vi "Get(X,Y)2.vi"(2 "[IN] index of (X,Y)":i32, 3 "[IN] Array coordi\nnates (X,Y) in Frame":dbl[](array[numeric])) -> (0 "[OUT] Y":dbl, 1 "[OUT] X":dbl)   [LabVIEW 2013]
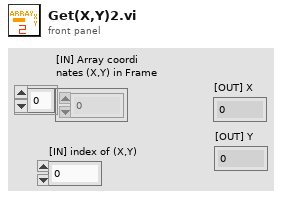
[diagram p1: front panel]
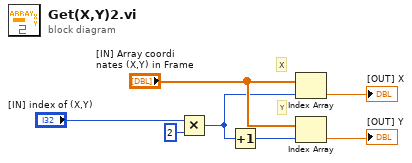
[diagram p0: block diagram]
diagram:
  # "Y"
  # "X"
  n1 = Multiply(x="[IN] index of (X,Y)", y=2) -> (x*y=w1:i32)
  n2 = Increment(x=w1) -> (x+1=w4:i32)
  n3 = Index Array(array="[IN] Array coordi\nnates (X,Y) in Frame", index=w1) -> (element=→"[OUT] X":dbl)
  n4 = Index Array(array="[IN] Array coordi\nnates (X,Y) in Frame", index=w4) -> (element=→"[OUT] Y":dbl)
